vi "io_write.vi"(6 "Block Logging (F)":bool, 8 "error in":errorcluster caption="error in (no error)", 10 "write buffer":string, 11 "VISA resource name":refnum<visa-resource-name>) -> (0 "error out":errorcluster, 3 "VISA resource name out":refnum<visa-resource-name>)   [LabVIEW 2020, in "Rohde&Schwarz RTx Oscilloscopes.lvlib" / "rsidr_core.lvlib"]
uses:
  rsidr_core.lvlib
  whitespace.ctl
  _type_Operation_Fgv_Debug.ctl
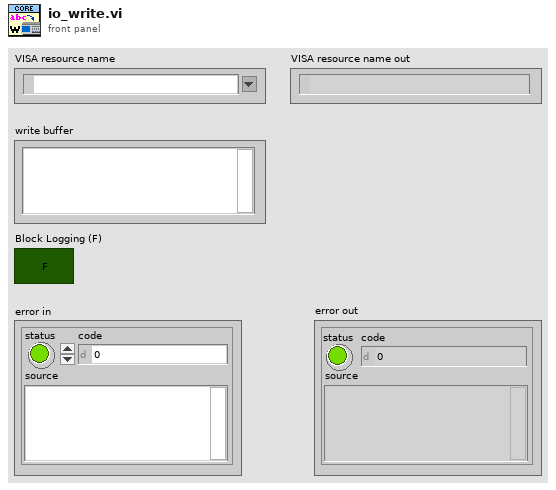
[diagram p1: front panel]
types:
  T1 = typedef "Rohde&Schwarz RTx Oscilloscopes.lvlib/rsidr_core.lvlib/_type_Operation_Fgv_Debug.ctl" = enum16{"Reset", "ReadCommand", "SetCommand"}
  T2 = typedef "Rohde&Schwarz RTx Oscilloscopes.lvlib/rsidr_core.lvlib/type_Session_Data.ctl" = cluster{"IDN string":string, "Instrument FW":string, "Instr type":string, "Instr type for err. msg.":string, "Installed Options":string[], "Ignore Error Messages":string, "Logging params":variant, "OPC Timeout":i32, "VISA Timeout":i32, "STB Poll VISA Timeout":i32, "Additional Flags":i32, "Wait Before Read":i32, "Wait Before Write":i32, "Option String Flags":i32, "IO Segment Size":i64, "VISA Access Mode":T3, "Interface Type":T4, "OPC Wait Mode":T5, "Bin Float Number  Format":T6, "Bin Integer Number Format":T7, "Simulate":bool, "VXIcapable":bool, "Duplicate Session":bool, "Add LF to Write":bool, "Logging":bool, "Fast Sweep":bool, "Query Instrument Status":bool, "Check Range":bool, "Check Options":bool, "OPC-sync Attr Writes":bool, "OPC-sync Attr Queries":bool}
  T3 = typedef "Rohde&Schwarz RTx Oscilloscopes.lvlib/rsidr_core.lvlib/type_VisaAccessMode.ctl" = u16
  T4 = typedef "Rohde&Schwarz RTx Oscilloscopes.lvlib/rsidr_core.lvlib/type_InterfaceType.ctl" = enum16{"Unknown", "GPIB", "VXI", "GPIB_VXI", "ASRL", "PXI", "TCPIP", "USB", "SOCKET"}
  T5 = typedef "Rohde&Schwarz RTx Oscilloscopes.lvlib/rsidr_core.lvlib/type_OPC_Wait_Mode.ctl" = enum16{"STBpolling", "STBpollingSlow", "STBpollingSuperSlow", "ServiceRequest", "OPCquery"}
  T6 = typedef "Rohde&Schwarz RTx Oscilloscopes.lvlib/rsidr_core.lvlib/type_Binary_Float_Number_Format.ctl" = enum16{"Float_4_Bytes_Swapped", "Float_4_Bytes", "Double_8_Bytes_Swapped", "Double_8_Bytes"}
  T7 = typedef "Rohde&Schwarz RTx Oscilloscopes.lvlib/rsidr_core.lvlib/type_Binary_Integer_Number_Format.ctl" = enum16{"Int32_4_Bytes_Swapped", "Int32_4 Bytes", "Int16_2_Bytes_Swapped", "Int16_2_Bytes"}
  T8 = typedef "whitespace.ctl" = u16
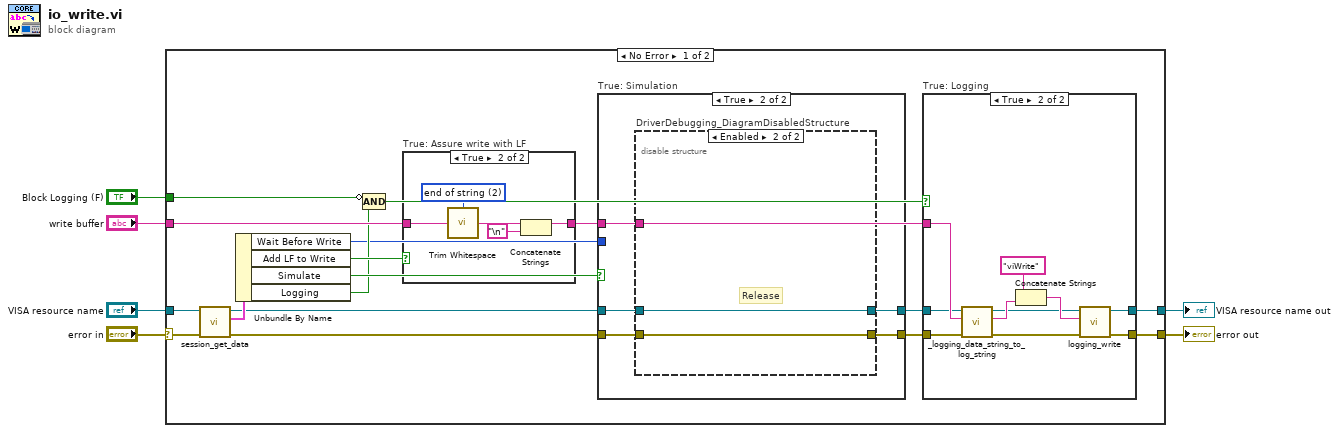
[diagram p0: block diagram]
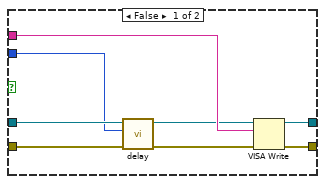
[diagram p3: hidden frame]
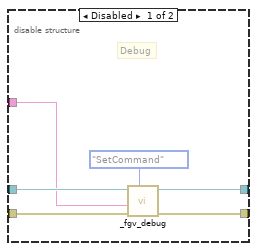
[diagram p4: hidden frame]
diagram:
  n1 = case shown="No Error" "error in" {
    selector: "error in" -> [w20 w64]
    tunnel: [w13 w63] -> w2
    tunnel: [w14 w64] -> w3
    tunnel: "write buffer" -> [w23 _]
    tunnel: "VISA resource name" -> [w19 w63]
    tunnel: "Block Logging (F)" -> [w7 _]
    frame No Error {
      n2 = call "session_get_data.vi"("error in"=w20, "VISA resource name"=w19) -> ("error out"=w18:errorcluster, "Session User Data out"=w21:T2, "VISA resource name out"=w10:refnum<visa-resource-name>)  [unwired: 6 in, 1 out]
      n3 = Unbundle By Name(w21) -> ("Wait Before Write"=w8:i32, "Add LF to Write"=w22:bool, "Simulate"=w17:bool, "Logging"=w16:bool)
      n4 = Compound Arithmetic op=AND(invert w7, w16) -> (w12:bool)
      n5 = case "True: Assure write with LF" shown="True" w22 {
        tunnel: w23 -> [w57 w60]
        tunnel: [w57 w62] -> w11
        frame False {
        }
        frame True {
          w58 = T8 2 items=["both", "start of string", "end of string"] ("location (both)")
          n6 = call "Trim Whitespace.vi"("string"=w60, "location (both)"=w58) -> ("trimmed string"=w59:string)
          n7 = Concatenate Strings(w59, "\n" ("Line Feed Constant")) -> (w62:string)
        }
      }
      n8 = case "True: Simulation" shown="True" w17 {
        tunnel: w18 -> [w42 w48]
        tunnel: w10 -> [w41 w47]
        tunnel: [w38 w46] -> w15
        tunnel: w11 -> [w43 w44]
        tunnel: [w37 w45] -> w9
        tunnel: w8 -> [w36 _]
        frame False {
          n9 = call "delay.vi"("error in"=w42, "Milliseconds to wait"=w36, "VISA resource name"=w41) -> ("error out"=w40:errorcluster, "VISA resource name out"=w39:refnum<visa-resource-name>)  [unwired: 7 in]
          n10 = VISA Write(VISA resource name=w39, write buffer=w43, error in (no error)=w40) -> (VISA resource name out=w37:refnum<visa-resource-name>, error out=w38:errorcluster)  [unwired: 1 out]
        }
        frame True {
          n11 = disable-structure "DriverDebugging_DiagramDisabledStructure" shown="Enabled" {
            disable-tunnel: w48 -> [w54 w55]
            disable-tunnel: [w52 w55] -> w46
            disable-tunnel: w47 -> [w53 w56]
            disable-tunnel: [w51 w56] -> w45
            disable-tunnel: w44 -> [w50 _]
            frame Disabled {
              # "Debug"
              n12 = call "_fgv_debug.vi"("Operation"=_type_Operation_Fgv_Debug."SetCommand", "error in"=w54, "Command in"=w50, "VISA resource name"=w53) -> ("error out"=w52:errorcluster, "VISA resource name out"=w51:refnum<visa-resource-name>)  [unwired: 6 in]
            }
            frame Enabled {
              # "Release"
            }
          }
        }
      }
      n13 = case "True: Logging" shown="True" w12 {
        tunnel: [w25 w34] -> w14
        tunnel: [w24 w33] -> w13
        tunnel: w15 -> [w25 w29]
        tunnel: w9 -> [w24 w28]
        tunnel: w11 -> [_ w35]
        frame False {
        }
        frame True {
          n14 = call "_logging_data_string_to_log_string.vi"("error in"=w29, "Raw string to log"=w35, "VISA resource name"=w28) -> ("error out"=w27:errorcluster, "Result log string"=w32:string, "VISA resource name out"=w26:refnum<visa-resource-name>)  [unwired: 6 in]
          n15 = Concatenate Strings("viWrite" ("format string"), w32) -> (w30:string)
          n16 = call "logging_write.vi"("error in"=w27, "String to write"=w30, "VISA resource name"=w26) -> ("error out"=w34:errorcluster, "VISA resource name out"=w33:refnum<visa-resource-name>)  [unwired: 7 in]
        }
      }
    }
    frame Error {
    }
  }
  "VISA resource name out" <- w2
  "error out" <- w3
